vi "getRowElements.vi"(8 "error in (no error)":errorcluster, 11 "Transaction in":refnum<class "Transaction.lvclass">) -> (0 "error out":errorcluster, 2 "Table Row":string[](array[string]), 3 "Transaction Out":refnum<class "Transaction.lvclass">)   [LabVIEW 2020, in "Transaction.lvclass"]
uses:
  Transaction.lvclass
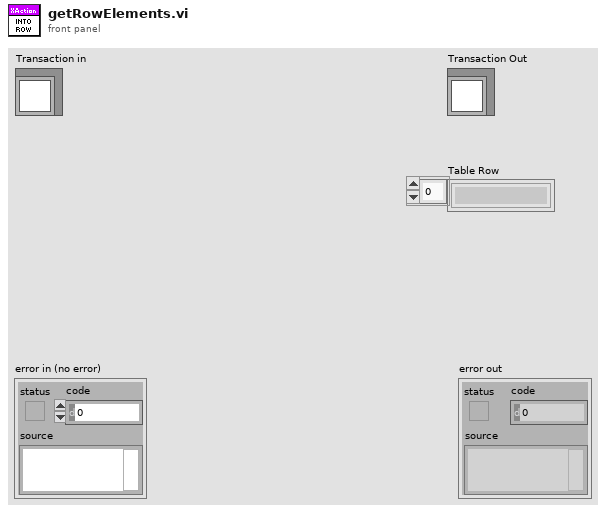
[diagram p1: front panel]
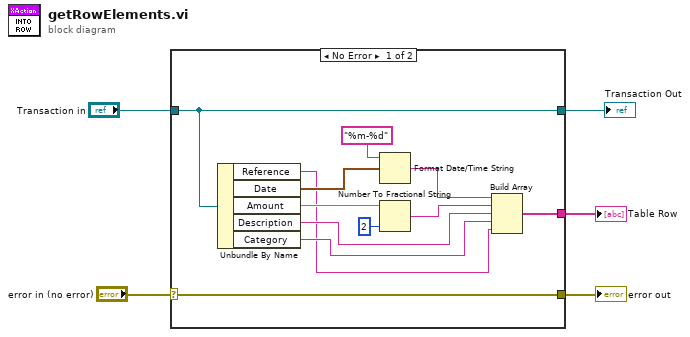
[diagram p0: block diagram]
diagram:
  n1 = case shown="No Error" "error in (no error)" {
    selector: "error in (no error)" -> [w17 w19]
    tunnel: [w17 w19] -> w4
    tunnel: "Transaction in" -> [w6 w18]
    tunnel: [w12 _] -> w3
    tunnel: [w6 w18] -> w1
    frame No Error {
      n2 = Unbundle By Name(w6) -> ("Reference"=w7:string, "Date"=w16:timestamp, "Amount"=w11:dbl, "Description"=w9:string, "Category"=w8:string)
      n3 = Format Date/Time String(time format string (%c)="%m-%d", seconds (now)=w16) -> (date/time string=w13:string)  [unwired: 1 in]
      n4 = Number To Fractional String(number=w11, precision (6)=i16 2) -> (F-format string=w10:string)  [unwired: 2 in]
      n5 = Build Array(w13, w10, w9, w8, w7) -> (w12:string[])
    }
    frame Error {
    }
  }
  "error out" <- w4
  "Table Row" <- w3
  "Transaction Out" <- w1
